vi "Find_maxima_params.vi"(0 "Array in":dbl[][](array[numeric]), 1 "Strip length":i32=600, 5 "Cursor.Cursor X":dbl, 7 "Cursor.Cursor Y":dbl, 9 "initial guess ROW":T1={"initial amplitude"=nan, "initial center"=nan, "initial std devi"=nan, "offset"=nan}, 11 "initial guess COL":T1={"initial amplitude"=nan, "initial center"=nan, "initial std devi"=nan, "offset"=nan}, 12 "Strip width":i32=20) -> (4 "Data and fits":dbl[][](array[numeric]), 6 "Slice":dbl[](array[numeric]), 8 "Params out":dbl[](array[numeric]), 10 "initial guess ROW ADJ 2":T1={"initial amplitude"=nan, "initial center"=nan, "initial std devi"=nan, "offset"=nan}, 15 "initial guess col  ADJ":T1={"initial amplitude"=nan, "initial center"=nan, "initial std devi"=nan, "offset"=nan})   [LabVIEW 2017]
panel:
  out "amplitude row":dbl
  out "center row":dbl
  out "standard deviation row":dbl
  out "amplitude col":dbl
  out "center  col":dbl
  out "standard deviation  col":dbl
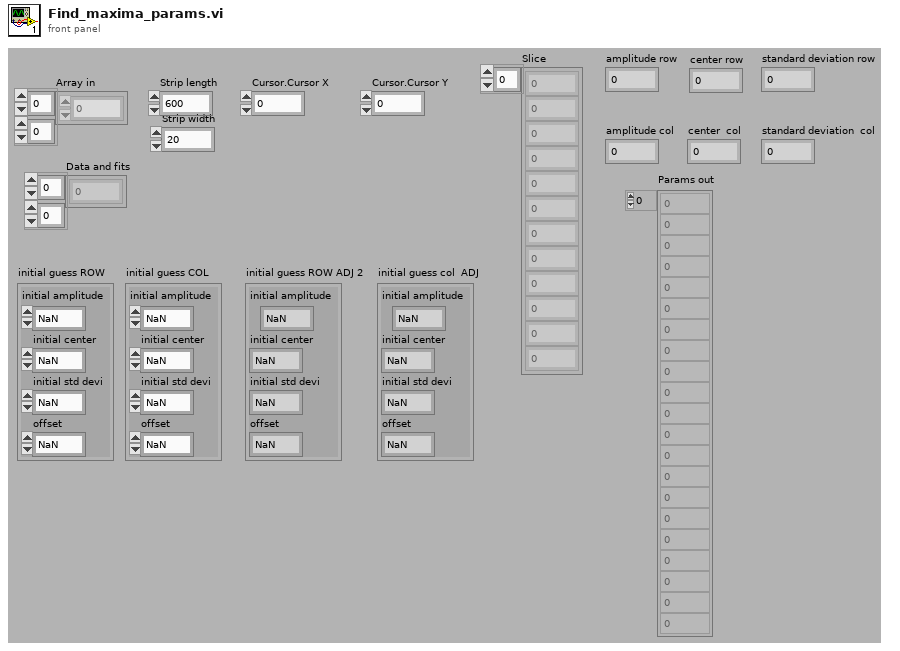
[diagram p1: front panel]
types:
  T1 = cluster{"initial amplitude":dbl, "initial center":dbl, "initial std devi":dbl, "offset":dbl}
  T2 = cluster{"initial amplitude":dbl, "initial center":dbl, "initial standard deviation":dbl, "offset":dbl}
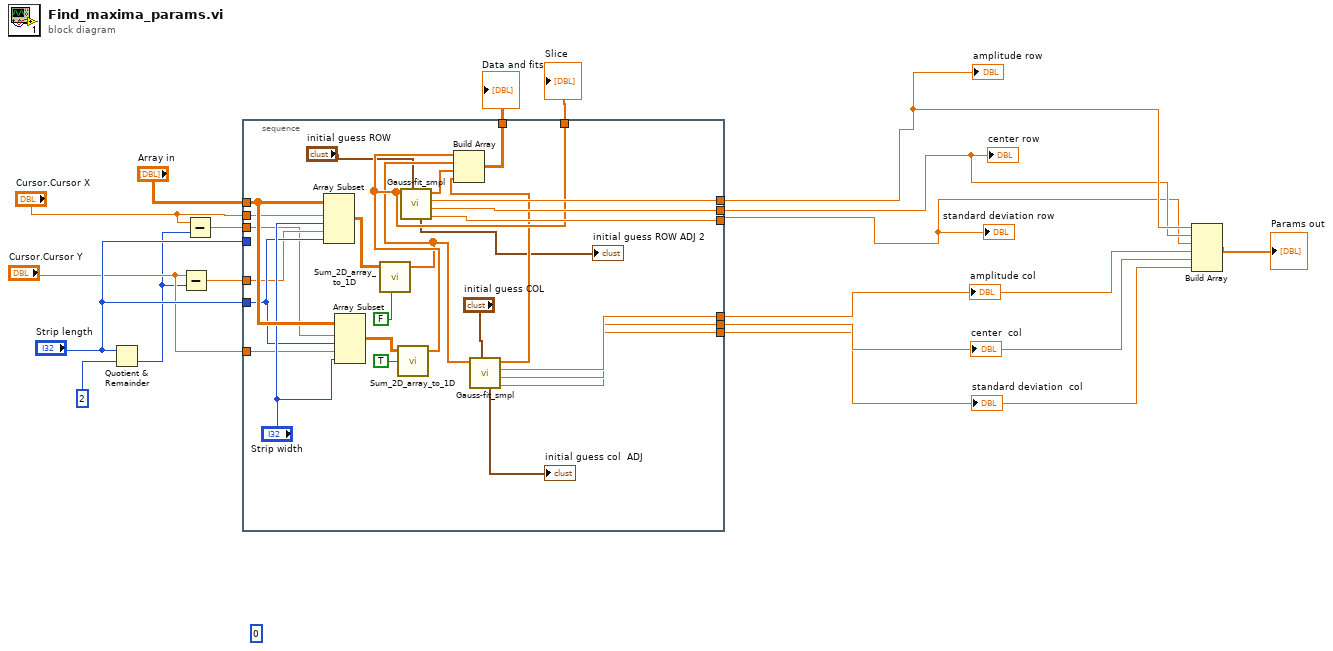
[diagram p0: block diagram]
diagram:
  (unwired) 0
  n1 = Quotient & Remainder(x="Strip length", y=2) -> (floor(x/y)=w2:i32)  [unwired: 1 out]
  n2 = Subtract(x="Cursor.Cursor Y", y=w2) -> (x-y=w6:dbl)
  n3 = Subtract(x="Cursor.Cursor X", y=w2) -> (x-y=w1:dbl)
  n4 = stacked-sequence {
    tunnel: "Array in" -> [w43]
    tunnel: "Cursor.Cursor X" -> [w37]
    tunnel: w6 -> [w21]
    tunnel: [w36] -> w13
    tunnel: [w35] -> w12
    tunnel: [w33] -> w15
    tunnel: [w34] -> w11
    tunnel: [w28] -> w10
    tunnel: [w27] -> w9
    tunnel: [w26] -> w8
    tunnel: [w25] -> w17
    tunnel: "Strip length" -> [w22]
    tunnel: "Strip length" -> [_]
    tunnel: "Cursor.Cursor Y" -> [w20]
    tunnel: w1 -> [w19]
    frame #0 {
      n5 = Array Subset(array=w43, index (row)=w37, length (row)="Strip width", index (col)=w21, length (col)=w22) -> (w42:dbl[][])
      n6 = Array Subset(array=w43, index (row)=w19, length (row)=w22, index (col)=w20, length (col)="Strip width") -> (w41:dbl[][])
      n7 = call <userlib>:"Sum_2D_array_to_1D.vi"("Cols/rows?"=FALSE, "Array in"=w42) -> ("Array summed"=w30:dbl[])  [unwired: 2 in, 1 out]
      n8 = call <userlib>:"Sum_2D_array_to_1D.vi"("Cols/rows?"=TRUE, "Array in"=w41) -> ("Array summed"=w33:dbl[])  [unwired: 2 in, 1 out]
      n9 = call <userlib>:"Gauss-fit_smpl.vi"("initial guess"="initial guess ROW", "FF array"=w33) -> ("standard deviation"=w34:dbl, "center"=w35:dbl, "amplitude"=w36:dbl, "Best fit array"=w32:dbl[], "initial guess ADJ"=→"initial guess ROW ADJ 2":T2)  [unwired: 4 in]
      n10 = call <userlib>:"Gauss-fit_smpl.vi"("initial guess"="initial guess COL", "FF array"=w30) -> ("standard deviation"=w26:dbl, "center"=w27:dbl, "amplitude"=w28:dbl, "Best fit array"=w29:dbl[], "initial guess ADJ"=→"initial guess col  ADJ":T2)  [unwired: 4 in]
      n11 = Build Array(w33, w30, w32, w29) -> (w25:dbl[][])
    }
  }
  "Data and fits" <- w17
  "standard deviation  col" <- w8
  "center  col" <- w9
  "amplitude col" <- w10
  "standard deviation row" <- w11
  "Slice" <- w15
  "center row" <- w12
  "amplitude row" <- w13
  n12 = Build Array(w13, w12, w11, w10, w9, w8) -> (→"Params out":dbl[])
